vi "Read Boiler Controller Constants.vi"(8 "error in":errorcluster, 11 "CFG File Refnum in":T2) -> (0 "error out":errorcluster, 2 "Controller Configuration":T1, 3 "CFG File Refnum out":T2)   [LabVIEW 2022 SP3]
uses:
  <vilib>/Utility/config.llb/Config Data RefNum.ctl
  Controller/Controller Configuration.ctl
  Boiler System Globals.vi
  <vilib>/Utility/config.llb/Read Key (U32).vi
  <vilib>/Utility/error.llb/Error Cluster From Error Code.vi
  <vilib>/ErrorRing/Error Ring.xnode
  <vilib>/Utility/config.llb/NI_LVConfig.lvlib
  Controller/Controller.lvlib
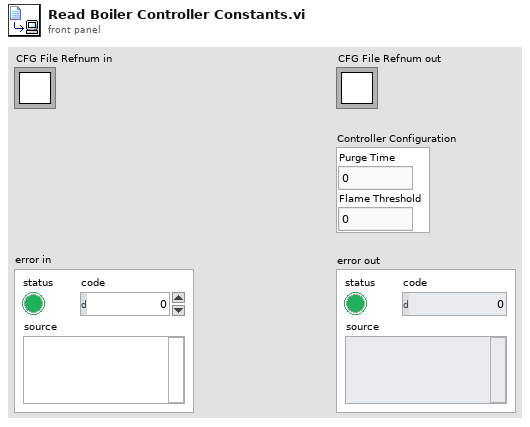
[diagram p1: front panel]
types:
  T1 = typedef "Controller.lvlib/Controller Configuration.ctl" = cluster{"Purge Time":u32, "Flame Threshold":u32}
  T2 = typedef "NI_LVConfig.lvlib/Config Data RefNum.ctl" = refnum<k1>
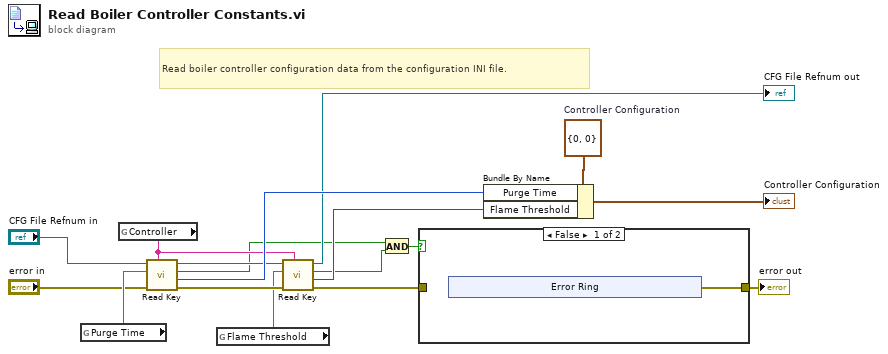
[diagram p0: block diagram]
diagram:
  w16 = T1 {"Purge Time"=0, "Flame Threshold"=0}  # Controller Configuration
  # "Read boiler controller configuration data from the configuration INI file."
  n1 = global read "Boiler System Globals.vi" "Purge Time"() -> (w13:string)
  n2 = global read "Boiler System Globals.vi" "Controller"() -> (w9:string)
  n3 = call-poly <vilib>:"Read Key.vi"("section"=w9, "error in (no error)"="error in", "key"=w13, "refnum"="CFG File Refnum in") -> ("error out"=w12:errorcluster, "value"=w17:u32, "found?"=w3:bool, "refnum out"=w8:T2)  [unwired: 4 in]
  n4 = global read "Boiler System Globals.vi" "Flame Threshold"() -> (w10:string)
  n5 = call-poly <vilib>:"Read Key.vi"("section"=w9, "error in (no error)"=w12, "key"=w10, "refnum"=w8) -> ("error out"=w11:errorcluster, "value"=w6:u32, "found?"=w4:bool, "refnum out"=→"CFG File Refnum out":T2)  [unwired: 4 in]
  n6 = And(x=w3, y=w4) -> (x .and. y?=w5:bool)
  n7 = case shown="False" w5 {
    tunnel: [w18 w24] -> w2
    tunnel: w11 -> [_ w24]
    frame False {
      n8 = xnode "Error Ring"() -> ("error out"=w18:errorcluster)
    }
    frame True {
    }
  }
  "error out" <- w2
  n9 = Bundle By Name(cluster=w16, "Purge Time"=w17, "Flame Threshold"=w6) -> (→"Controller Configuration":T1)
